vi "QueryLossDialog.vi"() -> (0 "drop?":bool, 1 "频率（KHz） 2":dbl=1.0 format="%#.3f", 2 "射频出 2":string(combo)="COM1", 3 "射频进 2":string(combo)="A2")   [LabVIEW 2015]
uses:
  Global/Globalclient.vi
panel:
  in  "射频进64":string(combo)="A1" caption="射频进"
  in  "Cancel":bool
  in  "OK":bool
  in  "频率（MHz）":dbl=600.0 min=600.0 max=3900.0 format="%#.3f"
  in  "射频出":string(combo)="COM1"
  in  "射频进128":string(combo)="A1" caption="射频进"
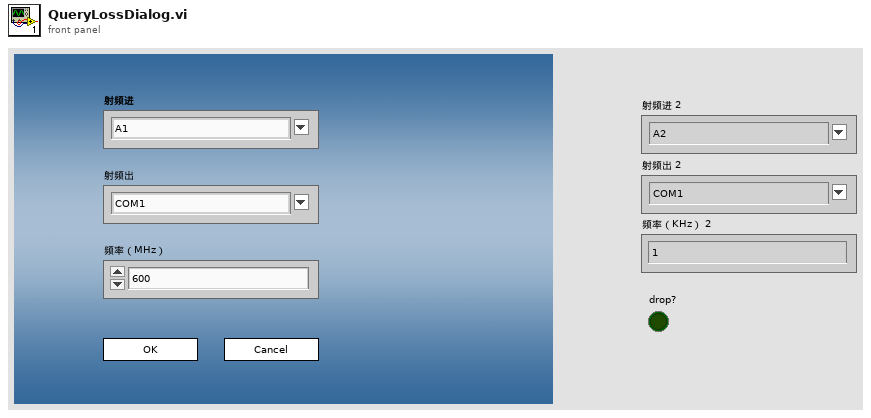
[diagram p1: front panel]
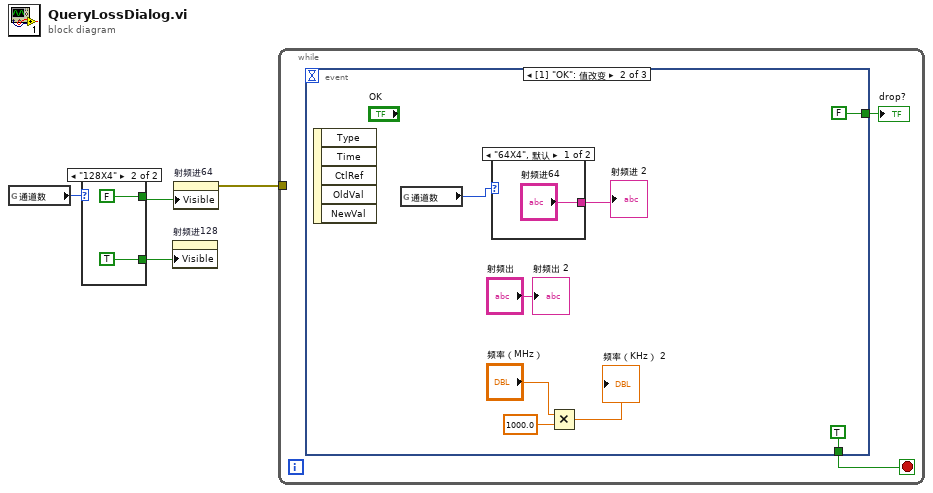
[diagram p0: block diagram]
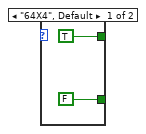
[diagram p2: hidden frame]
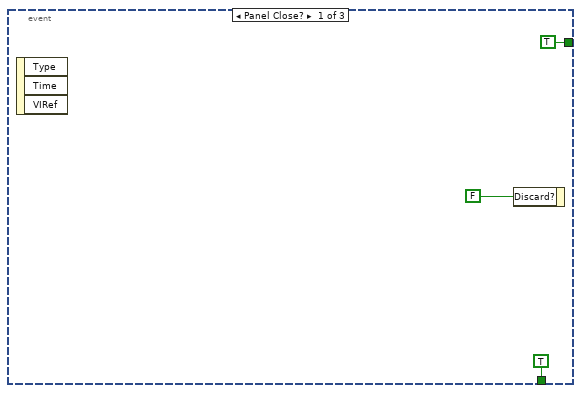
[diagram p3: hidden frame]
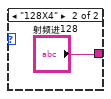
[diagram p4: hidden frame]
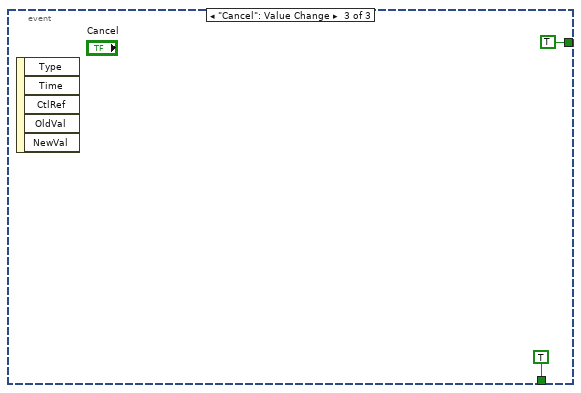
[diagram p5: hidden frame]
diagram:
  n1 = global read "Globalclient.vi" "通道数"() -> (w4:enum16{"64X4", "128X4"})
  n2 = case shown="\"128X4\"" w4 {
    tunnel: [FALSE ("可见") TRUE ("可见")] -> w3
    tunnel: [TRUE ("可见") FALSE ("可见")] -> w2
    frame "64X4", Default {
    }
    frame "128X4" {
    }
  }
  n3 = property on="射频进128" class="CmbBox"("Visible"=w3) -> ()  [unwired: 2 in, 2 out]
  n4 = property on="射频进64" class="CmbBox"("Visible"=w2) -> (error out=w1:errorcluster)  [unwired: 2 in, 1 out]
  n5 = while {
    tunnel: w1 -> [_]
    stop <- w9 stop-if-true
    n6 = event shown="[1] \"OK\": 值改变" {
      selector: _ -> [_ _ _]
      dyn-events: _ -> [_ _ _]
      timeout: _ -> [_ _ _]
      tunnel: [TRUE FALSE TRUE] -> w10
      tunnel: [TRUE TRUE TRUE] -> w9
      event Panel Close? {
        n7 = event-data() -> ()  [unwired: 1 in, 3 out]
        n8 = event-data("Discard?"=FALSE ("放弃？")) -> ()  [unwired: 1 in, 1 out]
      }
      event "OK": Value Change {
        n9 = event-data() -> ()  [unwired: 1 in, 5 out]
        n10 = global read "Globalclient.vi" "通道数"() -> (w15:enum16{"64X4", "128X4"})
        n11 = case shown="\"64X4\", 默认" w15 {
          tunnel: ["射频进64" "射频进128"] -> w14
          frame "64X4", Default {
          }
          frame "128X4" {
          }
        }
        "射频进 2" <- w14
        n12 = Multiply(x="频率（MHz）", y=1000.0) -> (x*y=→"频率（KHz） 2":dbl)
        "射频出 2" <- "射频出"
      }
      event "Cancel": Value Change {
        n13 = event-data() -> ()  [unwired: 1 in, 5 out]
      }
    }
    "drop?" <- w10
  }
